vi "Convex Hull 3D (GiftWrap).vi"(0 "Vertices":sgl[][](array[numeric])) -> (1 "Convex hull triangles, indexed":T1[](array[typedef]), 2 "Stack error":errorcluster)   [LabVIEW 2014]
uses:
  Typedefs/Triangle, indexed.ctl
  Typedefs/Edge, indexed.ctl
  Subroutines/Cross product 3D.vi
  Subroutines/Unit vector.vi
panel:
  # "PN 29/03/2015"
  # "Vertices"
  # "Indices"
  # "Unit normal"
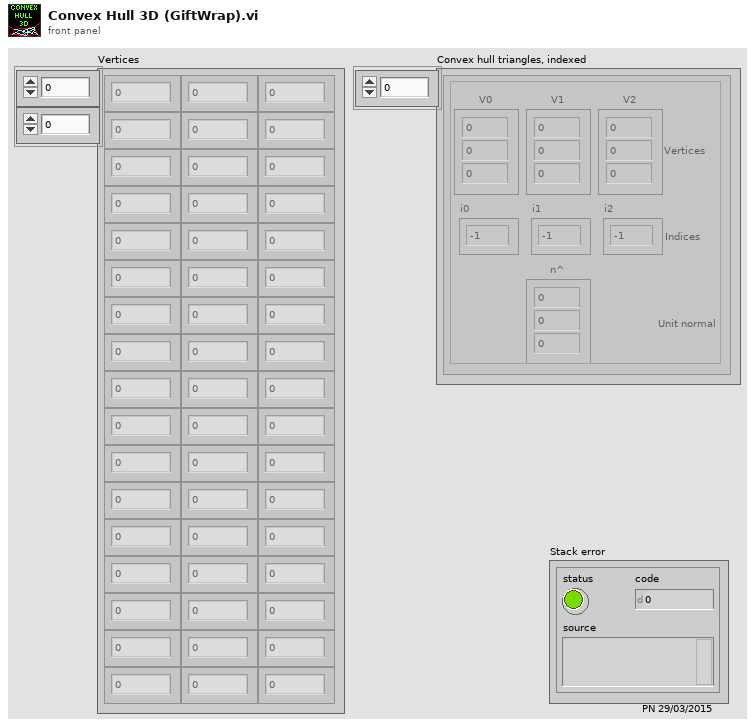
[diagram p1: front panel]
types:
  T1 = typedef "Triangle, indexed.ctl" = cluster{"V0":sgl[], "V1":sgl[], "V2":sgl[], "n^":sgl[], "i0":i32, "i1":i32, "i2":i32}
  T2 = typedef "Edge, indexed.ctl" = cluster{"V0":sgl[], "V1":sgl[], "i0":i32, "i1":i32}
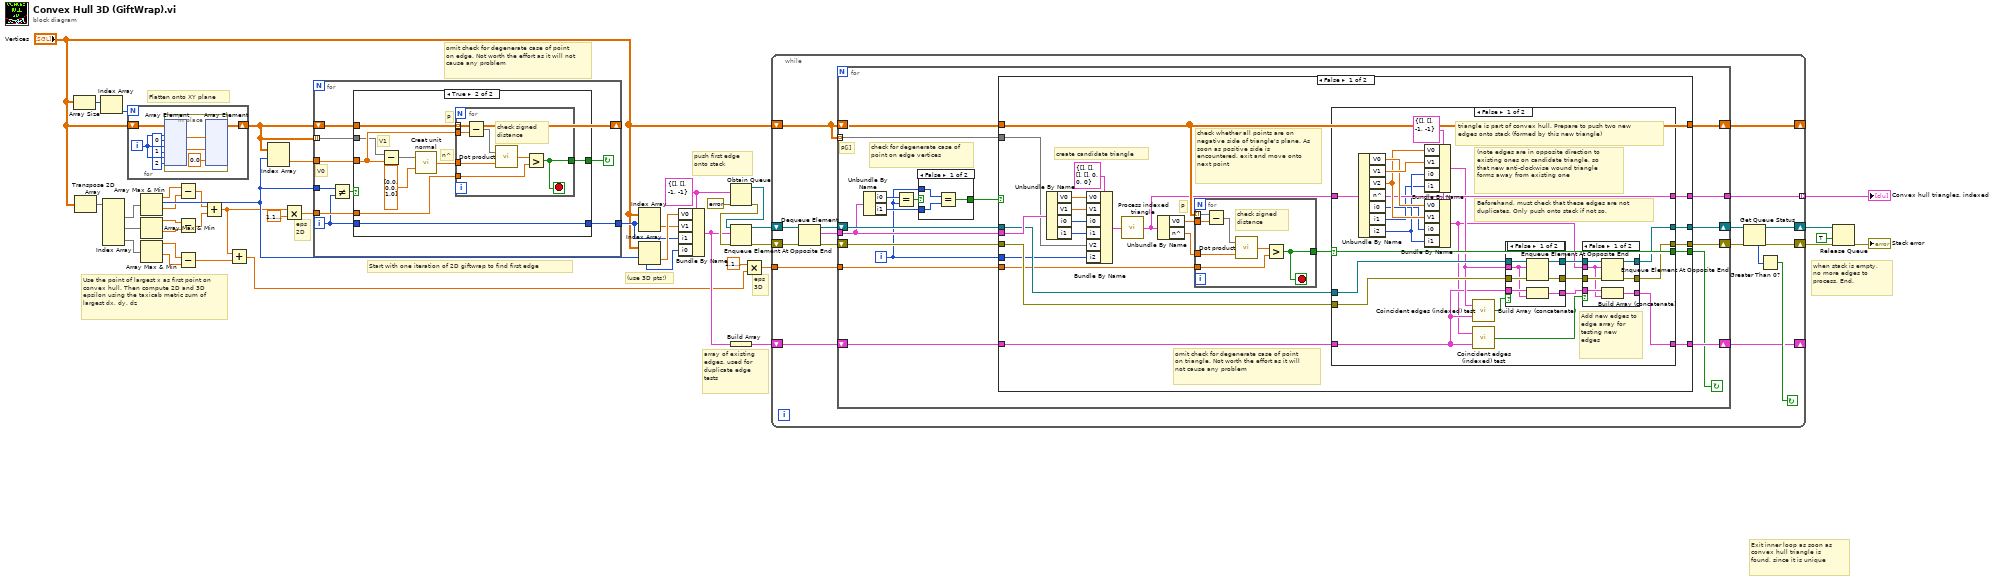
[diagram p0: block diagram]
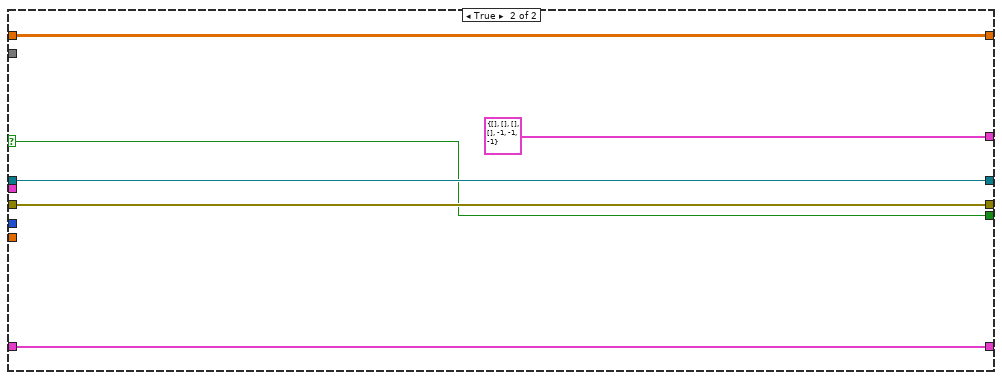
[diagram p6: hidden frame]
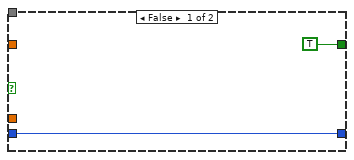
[diagram p7: hidden frame]
diagram:
  w34 = T2 {"V0"=[], "V1"=[], "i0"=-1, "i1"=-1} ("Edge, indexed")
  # "Use the point of largest x as first point on convex hull. Then compute 2D and 3D epsilon using the taxicab metric sum of largest dx, dy, dz"
  # "Flatten onto XY plane"
  # "Start with one iteration of 2D giftwrap to find first edge"
  # "eps 3D"
  # "array of existing edges, used for duplicate edge tests"
  # "omit check for degenerate case of point on edge. Not worth the effort as it will not cause any problem"
  # "when stack is empty, no more edges to process. End."
  # "Exit inner loop as soon as convex hull triangle is found, since it is unique"
  # "(use 3D pts!)"
  # "push first edge onto stack"
  # "eps 2D"
  n1 = Array Size(array="Vertices") -> (size(s)=w2:i32[])
  n2 = Transpose 2D Array(2D array="Vertices") -> (transposed array=w24:sgl[][])
  n3 = Index Array(array=w2) -> (element=w1:i32)  [unwired: 1 in]
  n4 = Index Array(array=w24) -> (element #1=w23:sgl[], element #2=w22:sgl[], element #3=w14:sgl[])  [unwired: 6 in]
  n5 = for {
    N: w1 -> [_]
    shift-right: [w46] -> w13
    shift-left: "Vertices" -> [w47]
    i -> [w45]
    n6 = in-place {
      n7 = in-place-array #1(w47, w45, 0, w45, 1, w45, 2) -> (w50:sgl, w49:sgl)  [unwired: 1 out]
      n8 = in-place-array #1(w50, w49, sgl 0.0 ("element")) -> (w46:sgl[][])  [unwired: 6 out]
    }
  }
  n9 = Array Max & Min(array=w23) -> (max value=w20:sgl, max index (indices)=w21:i32, min value=w19:sgl)  [unwired: 1 out]
  n10 = Array Max & Min(array=w22) -> (max value=w18:sgl, min value=w17:sgl)  [unwired: 2 out]
  n11 = Array Max & Min(array=w14) -> (max value=w16:sgl, min value=w15:sgl)  [unwired: 2 out]
  n12 = Subtract(x=w20, y=w19) -> (x-y=w12:sgl)
  n13 = Subtract(x=w18, y=w17) -> (x-y=w11:sgl)
  n14 = Subtract(x=w16, y=w15) -> (x-y=w10:sgl)
  n15 = Add(x=w12, y=w11) -> (x+y=w9:sgl)
  n16 = Add(x=w9, y=w10) -> (x+y=w5:sgl)
  n17 = Index Array(array=w13, index (row)=w21) -> (element=w41:sgl[])  [unwired: 1 in]
  n18 = Multiply(x=w9, y=sgl 1.1920929e-07) -> (x*y=w7:sgl)
  n19 = for {
    tunnel: w41 -> [w59]
    tunnel: w13 -> [w56] mode=indexing
    shift-right: [w57] -> _
    shift-left: w13 -> [w57]
    tunnel: w7 -> [w58]
    tunnel: [w53] -> w28
    tunnel: w21 -> [w51]
    i -> [w52]
    stop <- w55 continue-if-true
    # "V0"
    n20 = Not Equal?(x=w51, y=w52) -> (x != y?=w54:bool)
    n21 = case shown="True" w54 {
      tunnel: w59 -> [_ w68]
      tunnel: w58 -> [_ w67]
      tunnel: w57 -> [_ w66]
      tunnel: w56 -> [_ w65]
      tunnel: [TRUE w64] -> w55
      tunnel: w52 -> [w60 w62]
      tunnel: [w60 w62] -> w53
      frame False {
      }
      frame True {
        # "P"
        # "n^"
        # "V1"
        n22 = Subtract(x=w65, y=w68) -> (x-y=w63:sgl[])
        n23 = call "Creat unit normal.vi"("E2"=sgl[] [0.0, 0.0, 1.0], "E1"=w63) -> ("n^ = (E1 x E2) / ||E1 x E2||"=w69:sgl[])
        n24 = for {
          tunnel: w69 -> [w77]
          tunnel: w66 -> [w76] mode=indexing
          tunnel: w68 -> [w75]
          tunnel: w67 -> [w74]
          tunnel: [w73] -> w64
          stop <- w73 stop-if-true
          # "check signed distance"
          n25 = Subtract(x=w76, y=w75) -> (x-y=w72:sgl[])
          n26 = call "Dot product.vi"("B"=w77, "A"=w72) -> ("A . B"=w71:sgl)
          n27 = Greater?(x=w71, y=w74) -> (0:w73:bool)
        }
      }
    }
  }
  n28 = Index Array(array="Vertices", index (row)=w28) -> (element=w32:sgl[])  [unwired: 1 in]
  n29 = Index Array(array="Vertices", index (row)=w21) -> (element=w33:sgl[])  [unwired: 1 in]
  n30 = Bundle By Name(cluster=w34, "V0"=w33, "V1"=w32, "i1"=w28, "i0"=w21) -> (w26:T2)
  n31 = Obtain Queue(element data type=w34, error in (no error)=errorcluster {"status"=FALSE, "code"=0, "source"=""}) -> (queue out=w39:refnum<queue>, error out=w37:errorcluster)  [unwired: 3 in, 1 out]
  n32 = Enqueue Element At Opposite End(queue=w39, element=w26, error in (no error)=w37) -> (queue out=w30:refnum<queue>, error out=w31:errorcluster)  [unwired: 1 in, 1 out]
  n33 = Build Array(w26) -> (w25:T2[])
  n34 = Multiply(x=sgl 1.1920929e-07, y=w5) -> (x*y=w4:sgl)
  n35 = while {
    shift-right: [w89] -> _
    shift-left: "Vertices" -> [w91]
    shift-right: [w85] -> w36
    shift-left: w30 -> [w94]
    shift-right: [w83] -> w35
    shift-left: w31 -> [w93]
    tunnel: w4 -> [w90]
    tunnel: [w80] -> w27 mode=indexing
    shift-right: [w78] -> _
    shift-left: w25 -> [w79]
    stop <- w81 continue-if-true
    n36 = Dequeue Element(queue=w94, error in (no error)=w93) -> (queue out=w88:refnum<queue>, element=w92:T2, error out=w87:errorcluster)  [unwired: 1 in, 1 out]
    n37 = for {
      tunnel: w91 -> [w104] mode=indexing
      tunnel: w92 -> [w105]
      shift-right: [w111] -> w89
      shift-left: w91 -> [w112]
      tunnel: w90 -> [w103]
      shift-right: [w107] -> w86
      shift-left: w88 -> [w109]
      shift-right: [w106] -> w84
      shift-left: w87 -> [w108]
      tunnel: [w110] -> w80
      shift-right: [w101] -> w78
      shift-left: w79 -> [w102]
      i -> [w95]
      stop <- w100 continue-if-true
      # "P[i]"
      # "check for degenerate case of point on edge vertices"
      n38 = Unbundle By Name(w105) -> ("i0"=w99:i32, "i1"=w97:i32)
      n39 = Equal?(x=w99, y=w95) -> (x = y?=w98:bool)
      n40 = case shown="False" w98 {
        selector: w98 -> [_ w116]
        tunnel: w95 -> [w114 _]
        tunnel: w97 -> [w115 _]
        tunnel: [w113 w116] -> w96
        frame False {
          n41 = Equal?(x=w114, y=w115) -> (x = y?=w113:bool)
        }
        frame True {
        }
      }
      n42 = case shown="False" w96 {
        selector: w96 -> [_ w196]
        tunnel: w105 -> [w129 _]
        tunnel: w104 -> [w120 _]
        tunnel: w112 -> [w133 w199]
        tunnel: w103 -> [w122 _]
        tunnel: [w133 w199] -> w111
        tunnel: [w131 w196] -> w100
        tunnel: [w124 T1 {"V0"=[], "V1"=[], "V2"=[], "n^"=[], "i0"=-1, "i1"=-1, "i2"=-1} ("Triangle out")] -> w110
        tunnel: w109 -> [w128 w198]
        tunnel: w108 -> [w130 w197]
        tunnel: [w127 w198] -> w107
        tunnel: [w126 w197] -> w106
        tunnel: w102 -> [w123 w195]
        tunnel: [w121 w195] -> w101
        tunnel: w95 -> [w117 _]
        frame False {
          # "P"
          # "omit check for degenerate case of point on triangle. Not worth the effort as it will not cause any problem"
          # "check whether all points are on negative side of triangle's plane. As soon as positive side is encountered, exit and move onto next point"
          # "create candidate triangle"
          n43 = Unbundle By Name(w129) -> ("V0"=w138:sgl[], "V1"=w137:sgl[], "i0"=w119:i32, "i1"=w118:i32)
          n44 = Bundle By Name(cluster=T1 {"V0"=[], "V1"=[], "V2"=[], "n^"=[], "i0"=0, "i1"=0, "i2"=0} ("Triangle, indexed"), "V0"=w138, "V1"=w137, "i0"=w119, "i1"=w118, "V2"=w120, "i2"=w117) -> (w136:T1)
          n45 = call "Process indexed triangle.vi"("Triangle in (indexed)"=w136) -> ("Triangle out (indexed)"=w125:T1)
          n46 = Unbundle By Name(w125) -> ("V0"=w134:sgl[], "n^"=w135:sgl[])
          n47 = for {
            tunnel: w135 -> [w193]
            tunnel: w133 -> [w192] mode=indexing
            tunnel: w134 -> [w191]
            tunnel: w122 -> [w190]
            tunnel: [w189] -> w132
            stop <- w189 stop-if-true
            # "check signed distance"
            n48 = Subtract(x=w192, y=w191) -> (x-y=w188:sgl[])
            n49 = call "Dot product.vi"("B"=w193, "A"=w188) -> ("A . B"=w187:sgl)
            n50 = Greater?(x=w187, y=w190) -> (0:w189:bool)
          }
          n51 = case shown="False" w132 {
            selector: w132 -> [w161 w186]
            tunnel: [w161 w186] -> w131
            tunnel: w130 -> [w156 w184]
            tunnel: w128 -> [w158 w185]
            tunnel: [w157 w185] -> w127
            tunnel: [w155 w184] -> w126
            tunnel: w125 -> [w150 w183]
            tunnel: [w150 w183] -> w124
            tunnel: w123 -> [w142 w182]
            tunnel: [w148 w182] -> w121
            frame False {
              w154 = T2 {"V0"=[], "V1"=[], "i0"=-1, "i1"=-1} ("Edge, indexed")
              # "(note edges are in opposite direction to existing ones on candidate triangle, so that new anti-clockwise wound triangle forms away from existing one"
              # "Add new edges to edge array for testing new edges"
              # "Beforehand, must check that these edges are not duplicates. Only push onto stack if not so."
              # "triangle is part of convex hull. Prepare to push two new edges onto stack (formed by this new triangle)"
              n52 = Unbundle By Name(w150) -> ("V0"=w152:sgl[], "V1"=w153:sgl[], "V2"=w151:sgl[], "i0"=w145:i32, "i1"=w146:i32, "i2"=w147:i32)  [unwired: 1 out]
              n53 = Bundle By Name(cluster=w154, "V0"=w151, "V1"=w153, "i0"=w147, "i1"=w146) -> (w144:T2)
              n54 = Bundle By Name(cluster=w154, "V0"=w152, "V1"=w151, "i0"=w145, "i1"=w147) -> (w141:T2)
              n55 = call "Coincident edges (indexed) test.vi"("Existing edges (indexed)"=w142, "Candidate edge (indexed)"=w144) -> ("Edge already exists"=w143:bool)
              n56 = call "Coincident edges (indexed) test.vi"("Existing edges (indexed)"=w142, "Candidate edge (indexed)"=w141) -> ("Edge already exists"=w140:bool)
              n57 = case shown="False" w143 {
                tunnel: [w178 w181] -> w160
                tunnel: [w177 w180] -> w159
                tunnel: w158 -> [w176 w181]
                tunnel: w156 -> [w175 w180]
                tunnel: w144 -> [w173 _]
                tunnel: w142 -> [w174 w179]
                tunnel: [w172 w179] -> w149
                frame False {
                  n58 = Enqueue Element At Opposite End(queue=w176, element=w173, error in (no error)=w175) -> (queue out=w178:refnum<queue>, error out=w177:errorcluster)  [unwired: 1 in, 1 out]
                  n59 = Build Array (concatenate)(w174, w173) -> (w172:T2[])
                }
                frame True {
                }
              }
              n60 = case shown="False" w140 {
                tunnel: w160 -> [w168 w171]
                tunnel: w159 -> [w167 w170]
                tunnel: [w166 w171] -> w157
                tunnel: [w165 w170] -> w155
                tunnel: w141 -> [w163 _]
                tunnel: w149 -> [w164 w169]
                tunnel: [w162 w169] -> w148
                frame False {
                  n61 = Enqueue Element At Opposite End(queue=w168, element=w163, error in (no error)=w167) -> (queue out=w166:refnum<queue>, error out=w165:errorcluster)  [unwired: 1 in, 1 out]
                  n62 = Build Array (concatenate)(w164, w163) -> (w162:T2[])
                }
                frame True {
                }
              }
            }
            frame True {
              # "Triangle does not form the convex hull, do nothing and just move on to next point"
            }
          }
        }
        frame True {
        }
      }
    }
    n63 = Get Queue Status(queue=w86, error in (no error)=w84) -> (queue out=w85:refnum<queue>, error out=w83:errorcluster, # elements in queue=w82:i32)  [unwired: 1 in, 5 out]
    n64 = Greater Than 0?(x=w82) -> (x > 0?=w81:bool)
  }
  "Convex hull triangles, indexed" <- w27
  n65 = Release Queue(queue=w36, force destroy? (F)=TRUE, error in (no error)=w35) -> (error out=→"Stack error":errorcluster)  [unwired: 2 out]
